vi "uart单通道.vi"() -> ()   [LabVIEW 2014]
uses:
  <vilib>/Instr/_visa.llb/VISA Configure Serial Port (Instr).vi
panel:
  in  "字符串":string="1"
  in  "保存":bool=TRUE
  out "X":dbl[][](graph)=[[-0.13176]]
  out "串口正常？":bool=TRUE
  out "读取缓冲区 2":string
  out "读取缓冲区":string="ÿ"
  in  "波特率":u32=9600
  in  "串口":refnum<visa-resource-name>="COM3" caption="VISA资源名称"
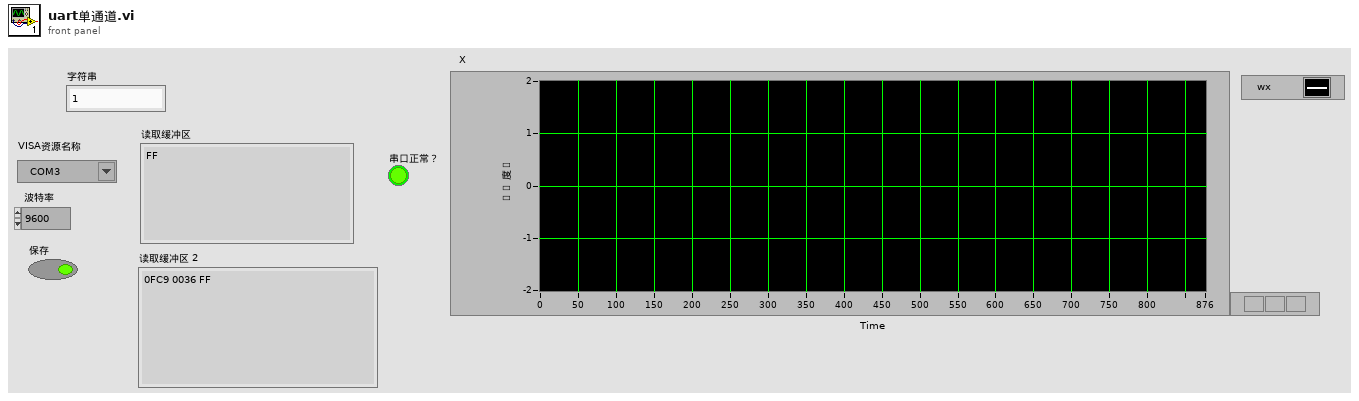
[diagram p1: front panel]
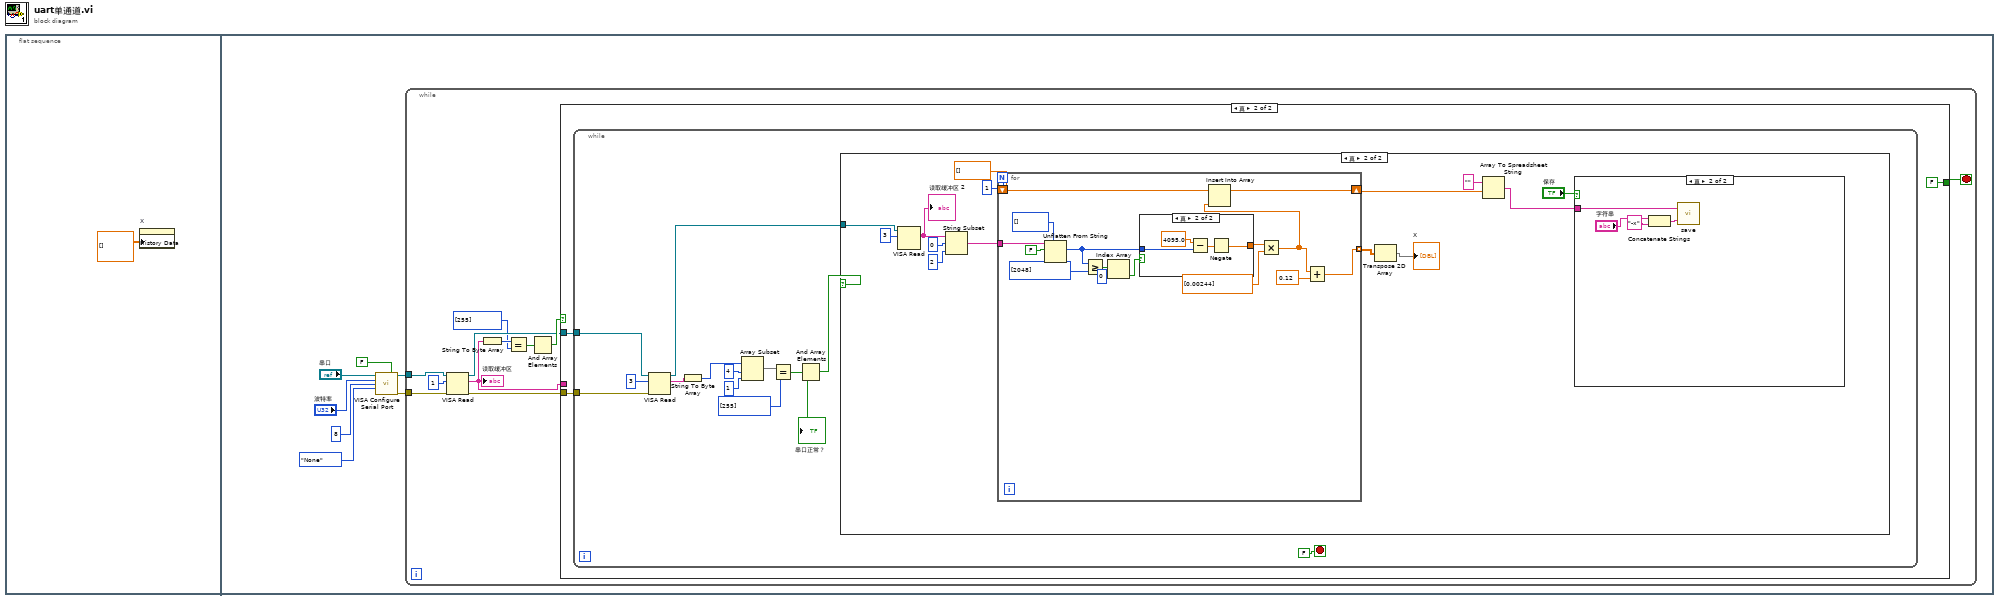
[diagram p0: block diagram]
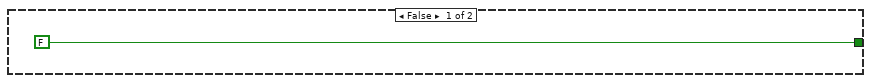
[diagram p2: hidden frame]
diagram:
  n1 = flat-sequence {
    frame #0 {
      n2 = property on="X" class="WFChart (严格)"("History Data"=dbl[][] [] ("历史数据")) -> ()  [unwired: 2 in, 2 out]
    }
    frame #1 {
      n3 = call-poly "VISA Configure Serial Port"("VISA resource name"="串口", "Enable Termination\nChar (T)"=FALSE ("Enable Termination\nChar (T)"), "baud rate (9600)"="波特率", "data bits (8)"=u16 8, "parity (0:none)"=enum16{"None", "Odd", "Even", "Mark", "Space"}."None") -> ("VISA resource name out"=w3:refnum<visa-resource-name>, "error out"=w2:errorcluster)  [unwired: 9 in]
      n4 = while {
        tunnel: w3 -> [w19]
        tunnel: w2 -> [w17]
        stop <- w9 stop-if-true
        n5 = VISA Read(VISA resource name=w19, byte count=u32 1 ("字节总数"), error in (no error)=w17) -> (VISA resource name out=w12:refnum<visa-resource-name>, read buffer=w13:string, error out=w11:errorcluster)  [unwired: 1 out]
        "读取缓冲区" <- w13
        n6 = String To Byte Array(string=w13) -> (unsigned byte array=w16:u8[])
        n7 = Equal?(x=w16, y=u8[] [255]) -> (x = y?=w15:bool[])
        n8 = And Array Elements(Boolean array=w15) -> (logical AND=w14:bool)
        n9 = case shown="真" w14 {
          tunnel: w13 -> [_ _]
          tunnel: w12 -> [_ w23]
          tunnel: w11 -> [_ w22]
          tunnel: [FALSE FALSE] -> w9
          frame False {
          }
          frame True {
            n10 = while {
              tunnel: w23 -> [w26]
              tunnel: w22 -> [w28]
              stop <- FALSE stop-if-true
              n11 = VISA Read(VISA resource name=w26, byte count=u32 3 ("字节总数"), error in (no error)=w28) -> (VISA resource name out=w24:refnum<visa-resource-name>, read buffer=w34:string)  [unwired: 2 out]
              n12 = String To Byte Array(string=w34) -> (unsigned byte array=w33:u8[])
              n13 = Array Subset(array=w33, index=4 ("索引"), length=1 ("长度")) -> (w29:u8[])
              n14 = Equal?(x=w29, y=u8[] [255]) -> (x = y?=w30:bool[])
              n15 = And Array Elements(Boolean array=w30) -> (logical AND=w25:bool)
              "串口正常？" <- w25
              n16 = case shown="真" w25 {
                tunnel: w24 -> [_ w45]
                frame False {
                }
                frame True {
                  n17 = VISA Read(VISA resource name=w45, byte count=u32 3 ("字节总数")) -> (read buffer=w46:string)  [unwired: 1 in, 3 out]
                  "读取缓冲区 2" <- w46
                  n18 = String Subset(string=w46, offset (0)=0 ("偏移量(0)"), length (rest)=2 ("长度（剩余）")) -> (substring=w48:string)
                  n19 = for {
                    N: 1 -> [_]
                    tunnel: w48 -> [w68]
                    shift-right: [w66] -> w38
                    shift-left: dbl[] [] -> [w67]
                    tunnel: [w55] -> w42 mode=indexing
                    n20 = Unflatten From String(type=i16[] [] ("无符号字节数组"), binary string=w68, data includes array or string size? (T)=FALSE ("数据中包含数组或字符串大小？(T)")) -> (value=w65:i16[])  [unwired: 2 in, 2 out]
                    n21 = Greater Or Equal?(x=w65, y=i16[] [2048]) -> (x >= y?=w62:bool[])
                    n22 = Index Array(array=w62, index=0 ("索引")) -> (element=w60:bool)
                    n23 = case shown="真" w60 {
                      tunnel: w65 -> [w70 w73]
                      tunnel: [w70 w71] -> w59
                      frame False {
                      }
                      frame True {
                        n24 = Subtract(x=4095.0, y=w73) -> (x-y=w72:dbl[])
                        n25 = Negate(x=w72) -> (-x=w71:dbl[])
                      }
                    }
                    n26 = Multiply(x=w59, y=dbl[] [0.00244]) -> (x*y=w56:dbl[])
                    n27 = Insert Into Array(array=w67, new element=w56) -> (w66:dbl[])  [unwired: 1 in]
                    n28 = Add(x=w56, y=0.12) -> (x+y=w55:dbl[])
                  }
                  n29 = Transpose 2D Array(2D array=w42) -> (transposed array=→"X":dbl[][])
                  n30 = Array To Spreadsheet String(array=w38, 3:"" ("格式字符串")) -> (spreadsheet string=w37:string)  [unwired: 1 in]
                  n31 = case shown="真" "保存" {
                    tunnel: w37 -> [_ w54]
                    frame False {
                    }
                    frame True {
                      n32 = Concatenate Strings("字符串", "-x" ("备注信息")) -> (w52:string)
                      n33 = call "save.vi"("备注信息"=w52, "data"=w54) -> ()
                    }
                  }
                }
              }
            }
          }
        }
      }
    }
  }
